vi "Test Subtract.vi"(8 "error in (no error)":errorcluster, 11 "Test Case In":refnum<class "Hi Res Arithm Test.lvclass">) -> (0 "error out":errorcluster, 3 "Test Case Out":refnum<class "Hi Res Arithm Test.lvclass">)   [LabVIEW 2021, in "Hi Res Arithm Test.lvclass"]
uses:
  Hi Res Arithm Test.lvclass
  Hi Res Arithm Test.lvclass/Hi Res Arithm Test.ctl
  4993e8ee-a06a-463a-9684-69129f64d5ce.vi
  High Res Arithmetic/High Res Arithmetic.lvclass
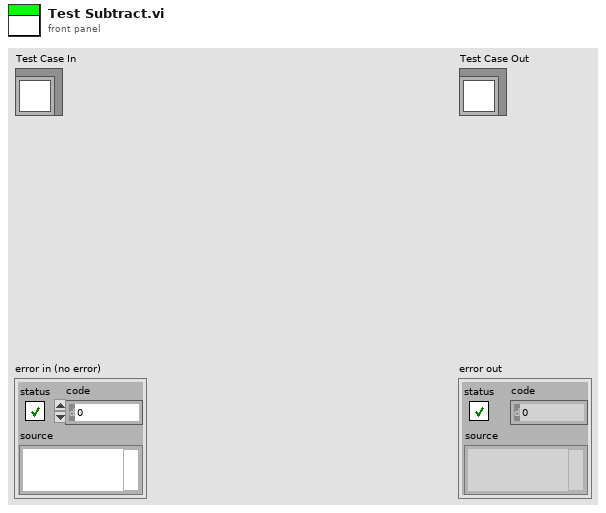
[diagram p1: front panel]
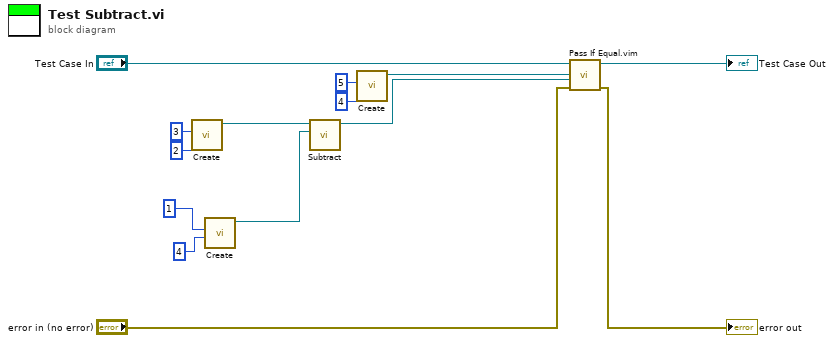
[diagram p0: block diagram]
diagram:
  n1 = call "Create.vi"("Denumerator"=i64 2, "Numerator"=i64 3 ("Integer Value")) -> ("Hi Res Arithm Test"=w9:refnum<class "High Res Arithmetic.lvclass">)  [unwired: 8 in, 1 out]
  n2 = call "Create.vi"("Denumerator"=i64 4 ("Integer Value"), "Numerator"=i64 1 ("Integer Value")) -> ("Hi Res Arithm Test"=w8:refnum<class "High Res Arithmetic.lvclass">)  [unwired: 8 in, 1 out]
  n3 = call "Subtract.vi"("High Res Arithmetic 2"=w8, "High Res Arithmetic 1"=w9) -> ("High Res Arithmetic sum"=w4:refnum<class "High Res Arithmetic.lvclass">)  [unwired: 8 in, 1 out]
  n4 = call "Create.vi"("Denumerator"=i64 4 ("Decimals"), "Numerator"=i64 5 ("Integer Value")) -> ("Hi Res Arithm Test"=w5:refnum<class "High Res Arithmetic.lvclass">)  [unwired: 8 in, 1 out]
  n5 = call "Pass If Equal.vim"("error in (no error)"="error in (no error)", "Actual"=w4, "Expected"=w5, "LUnit Test Case In"="Test Case In") -> ("error out"=→"error out":errorcluster, "LUnit Test Case Out"=→"Test Case Out":refnum<class "Hi Res Arithm Test.lvclass">)  [unwired: 6 in]
